vi "Get Tree Items.vi"(10 "Filter":T1, 11 "Result Model In":refnum<class "Result Model.lvclass">) -> (2 "Tree Items":T2(array[cluster]))   [LabVIEW 2020, in "Result Model.lvclass"]
uses:
  Result Model.lvclass
  Tree Item Filter.ctl
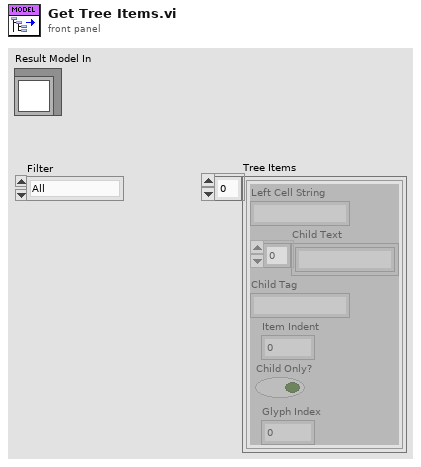
[diagram p1: front panel]
types:
  T1 = typedef "Result Model.lvclass/Tree Item Filter.ctl" = enum16{"All", "Only Fails"}
  T2 = cluster{"Left Cell String":string, "Child Text":string[], "Child Tag":string, "Item Indent":i32, "Child Only?":bool, "Glyph Index":i32}[]
  T3 = typedef "Result.lvlib/Status.ctl" = enum16{"", "Passed", "Failed", "Error", "Skipped", "Setup Error", "Broken", "Teardown Error"}
  T4 = cluster{"Left Cell String":string, "Child Text":string[], "Child Tag":string, "Item Indent":i32, "Child Only?":bool, "Glyph Index":i32}
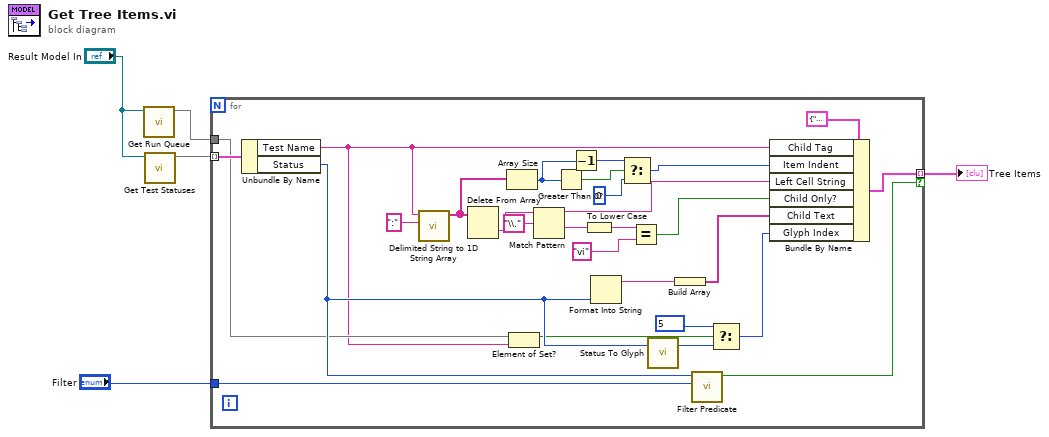
[diagram p0: block diagram]
diagram:
  n1 = call "Get Run Queue.vi"("Result Model in"="Result Model In") -> ("Run Queue"=w2:set{string})  [unwired: 10 in]
  n2 = call "Get Test Statuses.vi"("Result Model in"="Result Model In") -> ("Test Statuses"=w1:map{string, T3})  [unwired: 10 in]
  n3 = for {
    tunnel: w1 -> [w32] mode=indexing
    tunnel: [w31] -> w5 mode=indexing if=w11
    tunnel: w2 -> [w18]
    tunnel: "Filter" -> [w12]
    n4 = Unbundle By Name(w32) -> ("Test Name"=w17:string, "Status"=w21:T3)
    n5 = call <vilib>:"Delimited String to 1D String Array.vi"("delimiter"=":", "delimited string"=w17) -> ("string array"=w26:string[])  [unwired: 9 in]
    n6 = Delete From Array(array=w26) -> (deleted portion=w29:string)  [unwired: 2 in, 1 out]
    n7 = Array Size(array=w26) -> (size(s)=w9:i32)
    n8 = Element of Set?(10:w17, 11:w18) -> (3:w16:bool)
    n9 = Match Pattern(string=w29, regular expression="\\.") -> (before substring=w27:string, after substring=w25:string)  [unwired: 1 in, 2 out]
    n10 = Greater Than 0?(x=w9) -> (x > 0?=w10:bool)
    n11 = Decrement(x=w9) -> (x-1=w8:i32)
    n12 = To Lower Case(string=w25) -> (all lower case string=w22:string)
    n13 = Format Into String(w21) -> (resulting string=w20:string)  [unwired: 3 in, 1 out]
    n14 = Select(t=w8, s=w10, f=0) -> (s? t:f=w7:i32)
    n15 = Equal?(x=w22, y="vi") -> (x = y?=w23:bool)
    n16 = call "Status To Glyph.vi"("Status"=w21) -> ("Listbox Symbol Ring Constant"=w13:i32)  [unwired: 2 in]
    n17 = Build Array(w20) -> (w19:string[])
    n18 = call "Filter Predicate.vi"("Filter"=w12, "Status"=w21) -> ("Include?"=w11:bool)  [unwired: 9 in]
    n19 = Select(t=5 ("Listbox Symbol Ring Constant"), s=w16, f=w13) -> (s? t:f=w14:i32)
    n20 = Bundle By Name(cluster=T4 {"Left Cell String"="", "Child Text"=[], "Child Tag"="", "Item Indent"=0, "Child Only?"=FALSE, "Glyph Index"=0} ("Item"), "Child Tag"=w17, "Item Indent"=w7, "Left Cell String"=w27, "Child Only?"=w23, "Child Text"=w19, "Glyph Index"=w14) -> (w31:T4)
  }
  "Tree Items" <- w5
